vi "tpg361_on_off.vi"() -> ()   [LabVIEW 2019]
panel:
  in  "SETTING UNIT":enum16{"NO CHANGE", "OFF", "ON"}(ring)
  out "GAUGE  Status":string
  out "Overall Status":bool
  out "Acknowledgement Status":bool
  out "err_out":errorcluster
  out "tpg361_visa 2":refnum<visa-resource-name>
  in  "tpg361_b2r 2":u32
  in  "tpg361_delay 3":u32=500
  in  "tpg361_delay 2":u32=500
  in  "tpg361_b2r":u32
  in  "err_in":errorcluster
  in  "tpg361_delay":u32=500
  in  "tpg361_visa":refnum<visa-resource-name>
  # "Gauge status:\n1 = OFF\n2 = ON"
  # "VISA"
  # "DELAY"
  # "BYTE AT PORT"
  # "STATUS"
  # "ERROR"
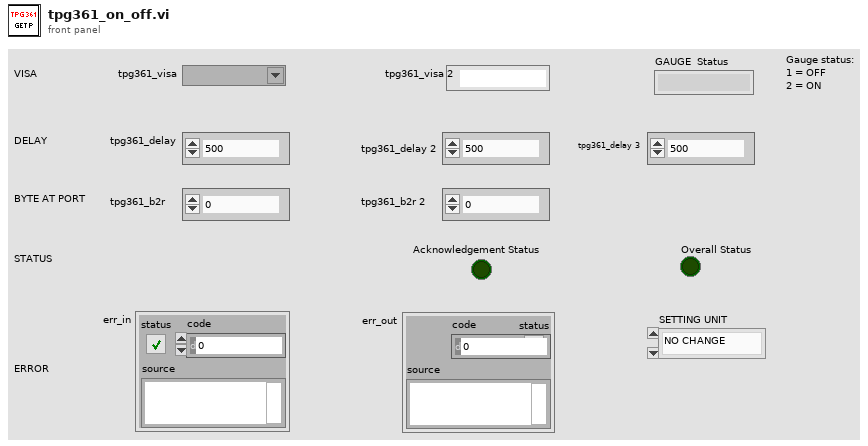
[diagram p1: front panel]
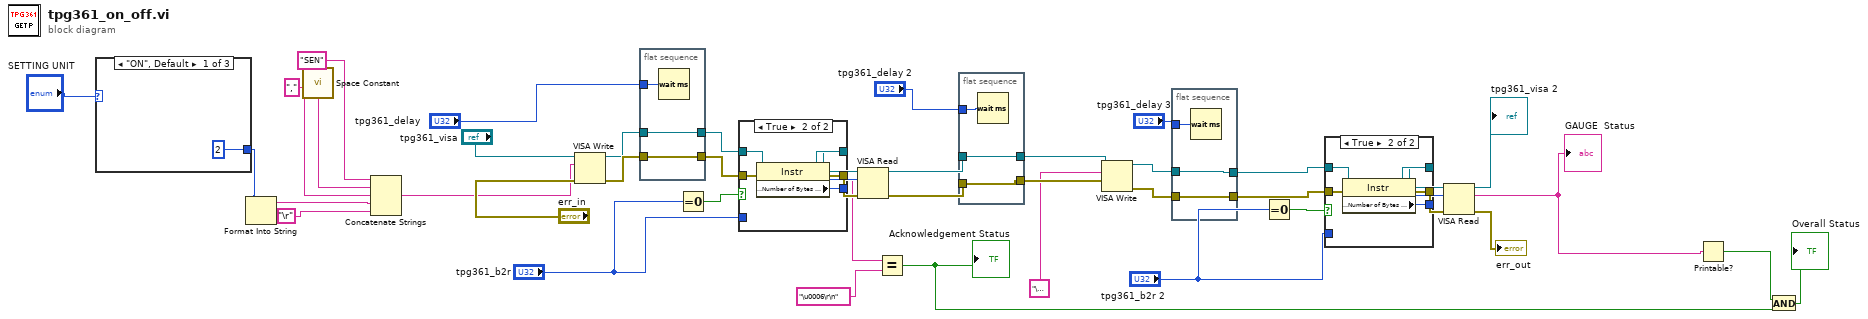
[diagram p0: block diagram]
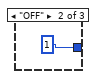
[diagram p2: hidden frame]
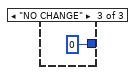
[diagram p3: hidden frame]
diagram:
  n1 = case shown="\"ON\", Default" "SETTING UNIT" {
    tunnel: [2 1 0] -> w4
    frame "ON", Default {
    }
    frame "OFF" {
    }
    frame "NO CHANGE" {
    }
  }
  n2 = Format Into String(w4) -> (resulting string=w2:string)  [unwired: 3 in, 1 out]
  n3 = call <vilib>:"Space Constant.vi"() -> ("String"=w5:string)
  n4 = Concatenate Strings("SEN" ("string"), w5, "," ("string"), w2, "\r") -> (w16:string)
  n5 = VISA Write(VISA resource name="tpg361_visa", write buffer=w16, error in (no error)="err_in") -> (VISA resource name out=w42:refnum<visa-resource-name>, error out=w44:errorcluster)  [unwired: 1 out]
  n6 = flat-sequence {
    tunnel: w44 -> [w49]
    tunnel: [w49] -> w43
    tunnel: w42 -> [w48]
    tunnel: [w48] -> w41
    tunnel: "tpg361_delay" -> [w50]
    frame #0 {
      n7 = Wait (ms)(milliseconds to wait=w50) -> ()  [unwired: 1 out]
    }
  }
  n8 = Equal To 0?(x="tpg361_b2r") -> (x = 0?=w37:bool)
  n9 = case shown="True" w37 {
    tunnel: w43 -> [w52 w58]
    tunnel: w41 -> [w53 w57]
    tunnel: [w53 w56] -> w35
    tunnel: [w52 w55] -> w34
    tunnel: [w51 w54] -> w33
    tunnel: "tpg361_b2r" -> [w51 _]
    frame False {
    }
    frame True {
      n10 = property class="Instr"(reference=w57, error in=w58) -> (reference out=w56:refnum<visa-resource-name>, error out=w55:errorcluster, "Serial Settings:Number of Bytes at Serial Port"=w54:u32)
    }
  }
  n11 = VISA Read(VISA resource name=w35, byte count=w33, error in (no error)=w34) -> (VISA resource name out=w32:refnum<visa-resource-name>, read buffer=w14:string, error out=w31:errorcluster)  [unwired: 1 out]
  n12 = Equal?(x=w14, y="\u0006\r\n") -> (x = y?=w10:bool)
  "Acknowledgement Status" <- w10
  n13 = flat-sequence {
    tunnel: [w59] -> w29
    tunnel: w32 -> [w61]
    tunnel: [w61] -> w30
    tunnel: "tpg361_delay 2" -> [w60]
    tunnel: w31 -> [w59]
    frame #0 {
      n14 = Wait (ms)(milliseconds to wait=w60) -> ()  [unwired: 1 out]
    }
  }
  n15 = VISA Write(VISA resource name=w30, write buffer="\u0005", error in (no error)=w29) -> (VISA resource name out=w22:refnum<visa-resource-name>, error out=w21:errorcluster)  [unwired: 1 out]
  n16 = flat-sequence {
    tunnel: [w63] -> w28
    tunnel: [w64] -> w27
    tunnel: w22 -> [w64]
    tunnel: w21 -> [w63]
    tunnel: "tpg361_delay 3" -> [w62]
    frame #0 {
      n17 = Wait (ms)(milliseconds to wait=w62) -> ()  [unwired: 1 out]
    }
  }
  n18 = Equal To 0?(x="tpg361_b2r 2") -> (x = 0?=w26:bool)
  n19 = case shown="True" w26 {
    tunnel: w28 -> [w66 w72]
    tunnel: w27 -> [w67 w71]
    tunnel: [w67 w70] -> w25
    tunnel: [w66 w69] -> w24
    tunnel: [w65 w68] -> w23
    tunnel: "tpg361_b2r 2" -> [w65 _]
    frame False {
    }
    frame True {
      n20 = property class="Instr"(reference=w71, error in=w72) -> (reference out=w70:refnum<visa-resource-name>, error out=w69:errorcluster, "Serial Settings:Number of Bytes at Serial Port"=w68:u32)
    }
  }
  n21 = VISA Read(VISA resource name=w25, byte count=w23, error in (no error)=w24) -> (VISA resource name out=→"tpg361_visa 2":refnum<visa-resource-name>, read buffer=w8:string, error out=→"err_out":errorcluster)  [unwired: 1 out]
  "GAUGE  Status" <- w8
  n22 = Printable?(1:w8) -> (0:w7:bool)
  n23 = And(x=w7, y=w10) -> (x .and. y?=→"Overall Status":bool)
